vi "ActionVIOnCompile.vi"(8 "error in (no error)":errorcluster, 11 "Device Item Ref in":T1 format="%.0x") -> (0 "error out":errorcluster)   [LabVIEW 2024, in "Embedded TDMS Logger System Explorer.lvlib"]
doc: "Collects the user defined System Definition of the Custom Device as defined in the System Explorer and compiles this into a transferrable format to send to the engine for execution."
uses:
  <vilib>/NI VeriStand/Custom Device API/Custom Device Item Ref.ctl
  Shared/Compiled.Settings.ctl
  Shared/SegmentOptions.ctl
  Shared/File Classes/File/FileAsCluster.ctl
  Shared/File Classes/Group/GroupAsCluster.ctl
  Shared/File Classes/Channel/ChannelAsCluster.ctl
  <vilib>/NI VeriStand/Custom Device API/Data Reference.ctl
  Shared/File Classes/Meta Data.ctl
  <vilib>/NI VeriStand/Custom Device API/Get Item Property (U16).vi
  <vilib>/NI VeriStand/Custom Device API/Get Item Property (Boolean).vi
  <vilib>/NI VeriStand/Custom Device API/Get Item Property (Double).vi
  <vilib>/NI VeriStand/Custom Device API/Set Item Property (Variant).vi
  Shared/File Classes/File/File.lvclass
  Embedded TDMS Logger System Explorer.lvlib
  <vilib>/NI VeriStand/Custom Device API/Custom Device API.lvlib
  <vilib>/NI/NIVS Inline Async API/_Data Access System Explorer/Data Access System Explorer.lvlib
  Shared/Embedded TDMS Logger Shared.lvlib
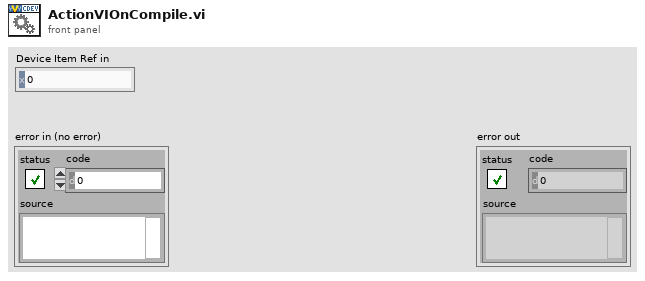
[diagram p1: front panel]
types:
  T1 = typedef "Custom Device API.lvlib/Custom Device Item Ref.ctl" = u64
  T2 = enum16{"Output/Write", "Input/Read", "Input/ReadWrite"}
  T3 = cluster{"Name":string, "Type":enum16{"Output/Write", "Input/Read", "Input/ReadWrite"}, "VS Refs":T1[]}
  T4 = typedef "Embedded TDMS Logger Shared.lvlib/Compiled.Settings.ctl" = cluster{"Name":string, "Async Init Timeout":u16, "Segment Files":bool, "Segment Every":dbl, "Segment by":T5, "dt per loop":dbl, "output cluster":T6}
  T5 = typedef "SegmentOptions.ctl" = enum16{"Time (s)", "Size (MB)"}
  T6 = typedef "FileAsCluster.ctl" = cluster{"Name":string, "Directory":string, "Date Captured":string, "Groups":T7[], "Meta Data":T10[], "File Start Time":timestamp, "appended path":path}
  T7 = typedef "GroupAsCluster.ctl" = cluster{"Name":string, "Channels":T8[], "Meta Data":T10[]}
  T8 = typedef "ChannelAsCluster.ctl" = cluster{"Name":string, "Data Reference":T9, "Wfm?":bool, "Decimation":i32, "Current Value":dbl, "Meta Data":T10[], "WfmPath":string}
  T9 = typedef "Custom Device API.lvlib/Data Reference.ctl" = i32
  T10 = typedef "Meta Data.ctl" = cluster{"Key":string, "Value":string}
  T11 = typedef "Custom Device API.lvlib/Custom Device Item Info.ctl" = cluster{"Name":string, "Is Channel":bool, "GUID":string, "Is Waveform":bool}
  T12 = cluster{"Name":string, "Type":enum16{"Output/Write", "Input/Read", "Input/ReadWrite"}, "VS Refs":T1[]}[]
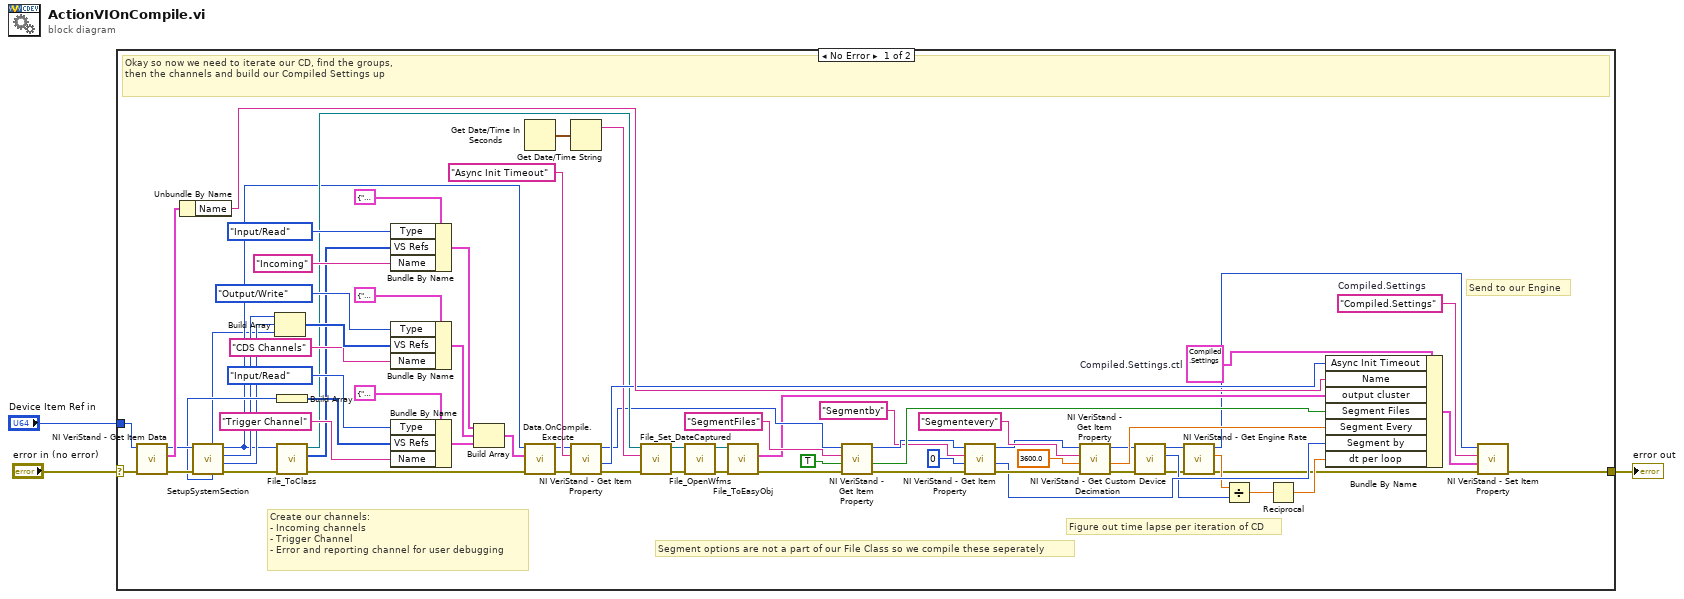
[diagram p0: block diagram]
diagram:
  n1 = case shown="No Error" "error in (no error)" {
    selector: "error in (no error)" -> [w71 w75]
    tunnel: [w72 w75] -> w3
    tunnel: "Device Item Ref in" -> [w66 _]
    frame No Error {
      w64 = T4 {"Name"="", "Async Init Timeout"=0, "Segment Files"=FALSE, "Segment Every"=0.0, "Segment by"=enum."Size (MB)", "dt per loop"=0.0, "output cluster"={"Name"="", "Directory"="", "Date Captured"="", "Groups"=[], "Meta Data"=[], "File Start Time"=timestamp(0 s since 1904-01-01), "appended path"=path ""}}  # Compiled.Settings.ctl
      w74 = "Compiled.Settings"  # Compiled.Settings
      # "Send to our Engine"
      # "Figure out time lapse per iteration of CD"
      # "Create our channels:\n- Incoming channels\n- Trigger Channel\n- Error and reporting channel for user debugging"
      # "Segment options are not a part of our File Class so we compile these seperately"
      # "Okay so now we need to iterate our CD, find the groups,\nthen the channels and build our Compiled Settings up"
      n2 = call <vilib>:"NI VeriStand - Get Item Data.vi"("error in (no error)"=w71, "Item Ref in"=w66) -> ("error out"=w37:errorcluster, "Item Info"=w70:T11, "Item Ref out"=w38:T1)  [unwired: 6 in, 1 out]
      n3 = Unbundle By Name(w70) -> ("Name"=w69:string)
      n4 = call "SetupSystemSection.vi"("error in (no error)"=w37, "Node Ptr"=w38) -> ("error out"=w22:errorcluster, "Error Code Ref"=w23:T1, "Triggered Ref"=w24:T1, "Parent Ref Out"=w10:T1, "Trigger Ref"=w25:T1, "Logging Ref"=w4:T1)  [unwired: 4 in]
      n5 = Build Array(w24, w23, w4) -> (w36:T1[])
      n6 = Build Array(w25) -> (w27:T1[])
      n7 = call "File_ToClass.vi"("error in (no error)"=w22, "Item Ref in"=w10) -> ("error out"=w14:errorcluster, "Channels"=w21:T1[], "File out"=w20:refnum<class "File.lvclass">)  [unwired: 7 in]
      n8 = Bundle By Name(cluster=T3 {"Name"="", "Type"=enum."Output/Write", "VS Refs"=[]} ("Group"), "Type"=T2."Input/Read", "VS Refs"=w21, "Name"="Incoming" ("Item Name")) -> (w31:T3)
      n9 = Bundle By Name(cluster=T3 {"Name"="", "Type"=enum."Output/Write", "VS Refs"=[]} ("Group"), "Type"=T2."Output/Write", "VS Refs"=w36, "Name"="CDS Channels") -> (w32:T3)
      n10 = Bundle By Name(cluster=T3 {"Name"="", "Type"=enum."Output/Write", "VS Refs"=[]} ("Group"), "Type"=T2."Input/Read", "VS Refs"=w27, "Name"="Trigger Channel") -> (w26:T3)
      n11 = Build Array(w31, w32, w26) -> (w47:T12)
      n12 = Get Date/Time In Seconds() -> (seconds since 1Jan1904=w65:timestamp)
      n13 = call <vilib>:"Data.OnCompile.Execute.vi"("error in"=w14, "VS Ref Groups"=w47, "Custom Device Ref"=w10) -> ("error out"=w13:errorcluster, "Custom Device Ref"=w9:T1)  [unwired: 7 in]
      n14 = Get Date/Time String(seconds (now)=w65) -> (date string=w19:string)  [unwired: 2 in, 1 out]
      n15 = call-poly <vilib>:"NI VeriStand - Get Item Property.vi"("error in (no error)"=w13, "Property Name"="Async Init Timeout", "Item Ref in"=w9) -> ("error out"=w15:errorcluster, "Value"=w67:u16, "Item Ref out"=w18:T1)  [unwired: 5 in, 1 out]
      n16 = call-dynamic "File_Set_DateCaptured.vi"("error in (no error)"=w15, "Date Captured"=w19, "File in"=w20) -> ("error out"=w5:errorcluster, "File out"=w8:refnum<class "File.lvclass">)  [unwired: 7 in]
      n17 = call-dynamic "File_OpenWfms.vi"("error in (no error)"=w5, "File in"=w8) -> ("error out"=w6:errorcluster, "File out"=w7:refnum<class "File.lvclass">)  [unwired: 8 in]
      n18 = call-dynamic "File_ToEasyObj.vi"("error in (no error)"=w6, "File in"=w7) -> ("error out"=w16:errorcluster, "output cluster"=w17:T6)  [unwired: 7 in, 1 out]
      n19 = call-poly <vilib>:"NI VeriStand - Get Item Property.vi"("error in (no error)"=w16, "Default Value"=TRUE, "Property Name"="SegmentFiles", "Item Ref in"=w18) -> ("error out"=w60:errorcluster, "Value"=w61:bool, "Item Ref out"=w59:T1)  [unwired: 4 in, 1 out]
      n20 = call-poly <vilib>:"NI VeriStand - Get Item Property.vi"("error in (no error)"=w60, "Default Value"=u16 0, "Property Name"="Segmentby", "Item Ref in"=w59) -> ("error out"=w54:errorcluster, "Value"=w51:u16, "Item Ref out"=w53:T1)  [unwired: 4 in, 1 out]
      n21 = call-poly <vilib>:"NI VeriStand - Get Item Property.vi"("error in (no error)"=w54, "Default Value"=3600.0, "Property Name"="Segmentevery", "Item Ref in"=w53) -> ("error out"=w40:errorcluster, "Value"=w52:dbl, "Item Ref out"=w39:T1)  [unwired: 4 in, 1 out]
      n22 = call <vilib>:"NI VeriStand - Get Custom Device Decimation.vi"("error in (no error)"=w40, "Device Ref in"=w39) -> ("error out"=w41:errorcluster, "Decimation"=w45:i32, "Device Ref out"=w42:T1)  [unwired: 7 in]
      n23 = call <vilib>:"NI VeriStand - Get Engine Rate.vi"("error in (no error)"=w41, "Item Ref in"=w42) -> ("error out"=w12:errorcluster, "Rate (Hz)"=w46:dbl, "Item Ref out"=w11:T1)  [unwired: 7 in]
      n24 = Divide(x=w46, y=w45) -> (x/y=w44:dbl)
      n25 = Reciprocal(x=w44) -> (1/x=w43:dbl)
      n26 = Bundle By Name(cluster=w64, "Async Init Timeout"=w67, "Name"=w69, "output cluster"=w17, "Segment Files"=w61, "Segment Every"=w52, "Segment by"=w51, "dt per loop"=w43) -> (w73:T4)
      n27 = call-poly <vilib>:"NI VeriStand - Set Item Property.vi"("error in (no error)"=w12, "Value"=w73, "Property Name"=w74, "Item Ref in"=w11) -> ("error out"=w72:errorcluster)  [unwired: 5 in, 2 out]
    }
    frame Error {
    }
  }
  "error out" <- w3
